vi "ModeLED.vi"(9 "Locate LED":bool, 10 "Choose Hue":bool) -> (2 "LED Mode":T1(ring))   [LabVIEW 2019]
uses:
  dsdata.vi
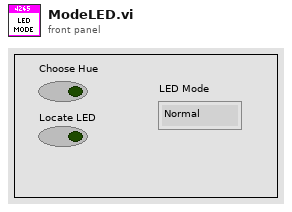
[diagram p1: front panel]
types:
  T1 = enum16{"Normal", "Party Mode", "Choose Hue", "Debug", "Locate LED"}
  T2 = enum16{"Center", "North", "NorthWest", "West", "SouthWest", "South", "SouthEast", "East", "NorthEast"}
  T3 = typedef "WPI_DriverStationRobotMode2.ctl" = enum16{"Autonomous Disabled", "Autonomous Enabled", "Teleop Disabled", "Teleop Enabled", "Disconnected", "Finish", "Test Disabled", "Test Enabled", "Emergency Stopped"}
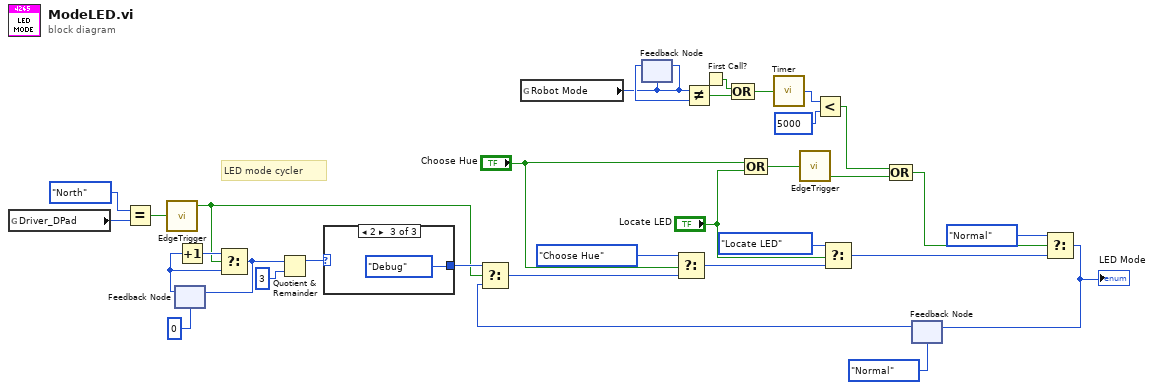
[diagram p0: block diagram]
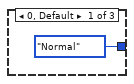
[diagram p2: hidden frame]
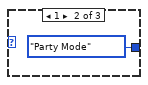
[diagram p3: hidden frame]
diagram:
  # "LED mode cycler"
  n1 = global read "dsdata.vi" "Driver_DPad"() -> (w12:T2)
  n2 = Equal?(x=T2."North", y=w12) -> (x = y?=w11:bool)
  n3 = call "EdgeTrigger.vi"("Input Signal"=w11) -> ("Rising Edge Trigger"=w3:bool)  [unwired: 2 out]
  n4 = feedback #1(0) -> (w8:i32)
  n5 = Increment(x=w8) -> (x+1=w9:i32)
  n6 = Select(t=w9, s=w3, f=w8) -> (s? t:f=w7:i32)
  n7 = feedback-in #1(w7) -> ()
  n8 = Quotient & Remainder(x=w7, y=3) -> (x-y*floor(x/y)=w5:i32)  [unwired: 1 out]
  n9 = case shown="2" w5 {
    tunnel: [T1."Normal" T1."Party Mode" T1."Debug"] -> w4
    frame 0, Default {
    }
    frame 1 {
    }
    frame 2 {
    }
  }
  n10 = global read "dsdata.vi" "Robot Mode"() -> (w32:T3)
  n11 = feedback #2(w32) -> (w33:T3)
  n12 = feedback-in #2(w32) -> ()
  n13 = Not Equal?(x=w32, y=w33) -> (x != y?=w16:bool)
  n14 = First Call?() -> (First Call?: T/F=w14:bool)
  n15 = Compound Arithmetic op=OR(w14, w16) -> (w15:bool)
  n16 = Compound Arithmetic op=OR("Choose Hue", "Locate LED") -> (w19:bool)
  n17 = call "Timer.vi"("Reset Timer"=w15) -> ("Time (ms)"=w28:u32)
  n18 = call "EdgeTrigger.vi"("Input Signal"=w19) -> ("Falling Edge Trigger"=w18:bool)  [unwired: 2 out]
  n19 = Less?(x=w28, y=u32 5000) -> (x < y?=w26:bool)
  n20 = Compound Arithmetic op=OR(w26, w18) -> (w25:bool)
  n21 = feedback #3(T1."Normal") -> (w1:T1)
  n22 = Select(t=w4, s=w3, f=w1) -> (s? t:f=w2:T1)
  n23 = Select(t=T1."Choose Hue", s="Choose Hue", f=w2) -> (s? t:f=w29:T1)
  n24 = Select(t=T1."Locate LED", s="Locate LED", f=w29) -> (s? t:f=w24:T1)
  n25 = Select(t=T1."Normal", s=w25, f=w24) -> (s? t:f=w17:T1)
  "LED Mode" <- w17
  n26 = feedback-in #3(w17) -> ()
